vi "Override Error Pointer.vi"(8 "error in (no error)":errorcluster, 10 "new error pointer":refnum<class "Error Pointer.lvclass">, 11 "Thread in":refnum<class "Thread.lvclass">) -> (0 "error out":errorcluster, 3 "Thread out":refnum<class "Thread.lvclass">)   [LabVIEW 2017, in "DSF Core.lvlib" / "Thread.lvclass"]
uses:
  Thread.lvclass
  Pointers/Error/Error Pointer.lvclass
  C:/Program Files (x86)/National Instruments/LabVIEW 2017/vi.lib/NI/Memory Manager/Classes/Pointer/Pointer.lvclass
  Thread.lvclass/Thread.ctl
  <vilib>/NI/Memory Manager/Classes/Pointer/Pointer.lvclass/Pointer.ctl
  <vilib>/NI/Memory Manager/Classes/Pointer/Get Address.vi
  <vilib>/NI/Memory Manager/Classes/Pointer/Get Internal.vi
  <vilib>/NI/Memory Manager/Classes/Pointer/Errors.vi
  <vilib>/NI/Memory Manager/Classes/Pointer/Zone.vi
  <vilib>/NI/Memory Manager/Classes/Pointer/Set Address.vi
  <vilib>/NI/Memory Manager/Classes/Pointer/Set Size.vi
  <vilib>/NI/Memory Manager/Classes/Pointer/Set Internal.vi
  <vilib>/NI/Memory Manager/Classes/Pointer/Check Null Pointer.vi
  <vilib>/NI/Memory Manager/Classes/Pointer/Create Error.vi
  <vilib>/NI/Memory Manager/Classes/Pointer/Null Pointer.vi
  <vilib>/NI/Memory Manager/Constants/Constants.vi
  <vilib>/NI/Memory Manager/Constants/Library Name.vi
  <vilib>/NI/Memory Manager/Classes/Pointer/Pointer Error Info.vi
  <vilib>/NI/Memory Manager/Constants/Pointer Class Name.vi
  <vilib>/NI/Memory Manager/VIs/New Error Cluster.vi
  <vilib>/NI/Memory Manager/VIs/New Error Cluster (512B).vi
  <vilib>/NI/Memory Manager/VIs/Set Error Status.vi
  <vilib>/NI/Memory Manager/VIs/Set Error Code.vi
  <vilib>/NI/Memory Manager/VIs/Set Error Source.vi
  <vilib>/NI/Memory Manager/VIs/Write String to Source.vi
  <vilib>/NI/Memory Manager/Classes/Pointer/Pointer.lvclass
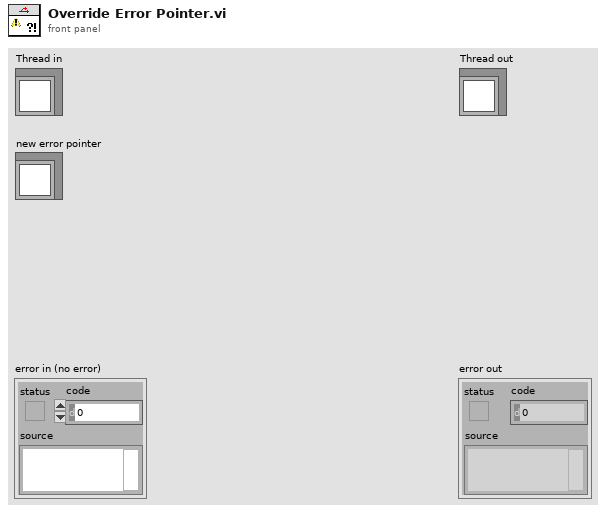
[diagram p1: front panel]
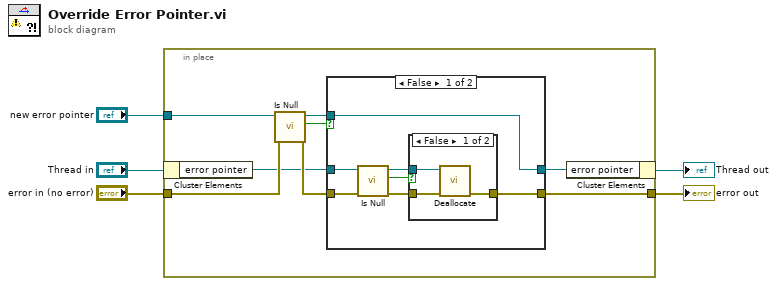
[diagram p0: block diagram]
diagram:
  n1 = in-place {
    in-place-border: "new error pointer" -> [w13]
    in-place-border: "error in (no error)" -> [w11]
    in-place-border: [w7] -> w1
    n2 = in-place-cluster #1("Thread in") -> ("error pointer"=w9:refnum<class "Error Pointer.lvclass">)
    n3 = call <vilib>:"Is Null.vi"("error in (no error)"=w11, "Pointer in"=w13) -> ("error out"=w10:errorcluster, "null?"=w12:bool, "Pointer out"=w8:refnum<class "Error Pointer.lvclass">)  [unwired: 7 in]
    n4 = case shown="False" w12 {
      tunnel: w9 -> [w17 w26]
      tunnel: w10 -> [w16 w25]
      tunnel: w8 -> [w14 _]
      tunnel: [w14 w26] -> w6
      tunnel: [w15 w25] -> w7
      frame False {
        n5 = call <vilib>:"Is Null.vi"("error in (no error)"=w16, "Pointer in"=w17) -> ("error out"=w18:errorcluster, "null?"=w19:bool, "Pointer out"=w20:refnum<class "Error Pointer.lvclass">)  [unwired: 7 in]
        n6 = case shown="False" w19 {
          tunnel: w20 -> [w21 _]
          tunnel: w18 -> [w22 w24]
          tunnel: [w23 w24] -> w15
          frame False {
            n7 = call <vilib>:"Deallocate.vi"("error in (no error)"=w22, "Pointer"=w21) -> ("error out"=w23:errorcluster)  [unwired: 8 in, 1 out]
          }
          frame True {
          }
        }
      }
      frame True {
      }
    }
    n8 = in-place-cluster #1("error pointer"=w6) -> (→"Thread out":refnum<class "Thread.lvclass">)
  }
  "error out" <- w1
